vi "ElevatorManual.vi"(8 "error in":errorcluster, 10 "Amount":dbl format="%#_13g", 11 "Direction":enum16{"Up", "Down"}(ring)) -> ()   [LabVIEW 2014, in "Elevator System.lvlib"]
uses:
  Elevator System.lvlib
  Typedef/MessageType.ctl
  Typedef/Commands.ctl
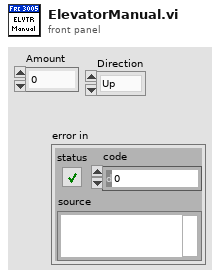
[diagram p1: front panel]
types:
  T1 = typedef "Elevator System.lvlib/MessageType.ctl" = cluster{"Name":T2, "Data":variant}
  T2 = typedef "Elevator System.lvlib/Commands.ctl" = enum16{"Home", "Stack", "Pickup", "Score", "Cycle", "Stop", "Manual Open", "Manual Close", "Manual Up", "Manual Down", "Gripper RC", "Gripper Cycle", "Wait On Gripper", "Wait On Elevator"}
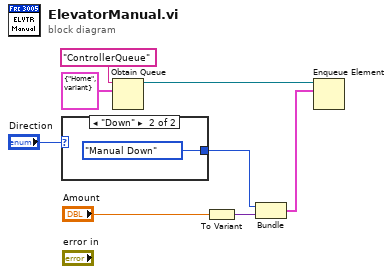
[diagram p0: block diagram]
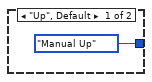
[diagram p2: hidden frame]
diagram:
  n1 = case shown="\"Down\"" "Direction" {
    tunnel: [Commands."Manual Up" ("Name") Commands."Manual Down" ("Name")] -> w2
    frame "Up", Default {
    }
    frame "Down" {
    }
  }
  n2 = Obtain Queue(name (unnamed)="ControllerQueue", element data type=T1 {"Name"=enum."Home", "Data"=variant} ("Message")) -> (queue out=w8:refnum<queue>)  [unwired: 3 in, 2 out]
  n3 = To Variant(anything="Amount") -> (Variant=w7:variant)
  n4 = Bundle("Name"=w2, "Variant"=w7) -> (w6:cluster{"Name":T2, "Variant":variant})  [unwired: 1 in]
  n5 = Enqueue Element(queue=w8, element=w6) -> ()  [unwired: 2 in, 3 out]
